vi "Post Build Script (manual build).vi"(7 "Project File Path":path, 8 "Package Source Folder":path=path "C:/user/patrick/git/Multichannel-Lockin/src", 9 "Package Version":string="2.8.9.18", 10 "Product Name":string="Multichannel Lockin", 11 "Output Package File Path":path) -> (0 "error out":errorcluster)   [LabVIEW 2019, in "PostBuildSupport.lvclass"]
doc: "After you manually build the Application and Installer inside your project, you can then call this VI to create single self-extracting installer file. It is meant to be placed inside \"Post-Build Custom Action.vi\" that is called post VIPM package build."
uses:
  PostBuildSupport.lvclass
  PostBuildSupport.lvclass/PostBuildSupport.ctl
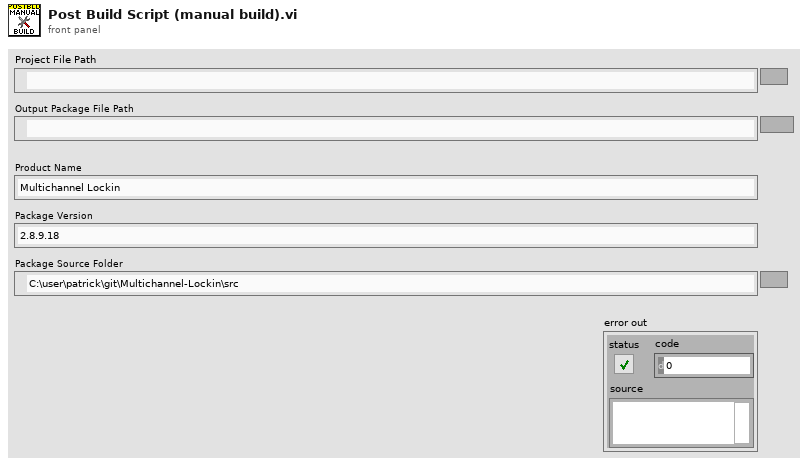
[diagram p1: front panel]
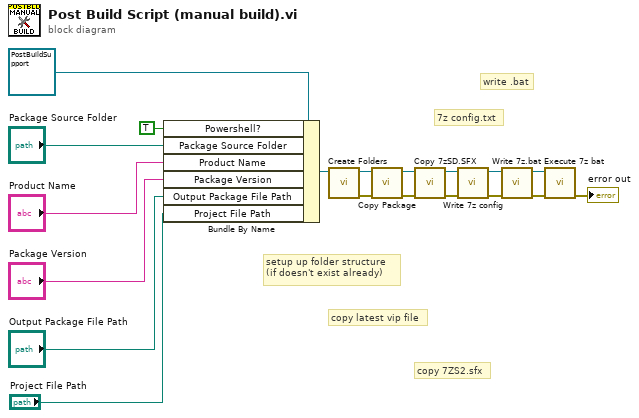
[diagram p0: block diagram]
diagram:
  # "copy 7ZS2.sfx"
  # "setup up folder structure \n(if doesn't exist already)"
  # "copy latest vip file"
  # "7z config.txt"
  # "write .bat"
  n1 = Bundle By Name(cluster=refnum<class "PostBuildSupport.lvclass"> refnum ("PostBuildSupport in"), "Powershell?"=TRUE, "Package Source Folder"="Package Source Folder", "Product Name"="Product Name", "Package Version"="Package Version", "Output Package File Path"="Output Package File Path", "Project File Path"="Project File Path") -> (w13:refnum<class "PostBuildSupport.lvclass">)
  n2 = call "Create Folders.vi"("PostBuildSupport in"=w13) -> ("error out"=w10:errorcluster, "PostBuildSupport out"=w15:refnum<class "PostBuildSupport.lvclass">)  [unwired: 9 in]
  n3 = call "Copy Package.vi"("error in (no error)"=w10, "PostBuildSupport in"=w15) -> ("error out"=w9:errorcluster, "PostBuildSupport out"=w14:refnum<class "PostBuildSupport.lvclass">)  [unwired: 8 in]
  n4 = call "Copy 7zSD.SFX.vi"("error in (no error)"=w9, "PostBuildSupport in"=w14) -> ("error out"=w11:errorcluster, "PostBuildSupport out"=w12:refnum<class "PostBuildSupport.lvclass">)  [unwired: 8 in]
  n5 = call "Write 7z config.vi"("error in (no error)"=w11, "PostBuildSupport in"=w12) -> ("error out"=w18:errorcluster, "PostBuildSupport out"=w19:refnum<class "PostBuildSupport.lvclass">)  [unwired: 8 in]
  n6 = call "Write 7z.bat.vi"("error in (no error)"=w18, "PostBuildSupport in"=w19) -> ("error out"=w7:errorcluster, "PostBuildSupport out"=w8:refnum<class "PostBuildSupport.lvclass">)  [unwired: 8 in]
  n7 = call "Execute 7z bat.vi"("error in (no error)"=w7, "PostBuildSupport in"=w8) -> ("error out"=→"error out":errorcluster)  [unwired: 8 in, 1 out]
